vi "Render Inverted Section with Null Array.vi"(8 "Error In":errorcluster) -> (0 "Error Out":errorcluster)   [LabVIEW 2018, in "Tests.lvlib" / "Render.lvlib"]
uses:
  Render.lvlib
  <vilib>/addons/_JKI Toolkits/Caraya/classes/Test/Test.lvclass
  <vilib>/addons/_JKI Toolkits/Caraya/classes/Assert/Assert.lvclass
  src/Toolkit/Toolkit.lvlib
  src/Toolkit/Low-Level/Support/Render to String.vi
  src/Toolkit/Low-Level/Support/Lex String.vi
  src/Toolkit/Data/Null/Null.lvclass
  src/Toolkit/Data/Array/Array.lvclass
  src/Toolkit/Data/Array/Support/From Data.vi
  src/Toolkit/Data/Pair/Pair.lvclass
  src/Toolkit/Data/Pair/Support/From Datum.vi
  src/Toolkit/Low-Level/Context/Compiler.lvclass
  D:/Users/cfield/Code/Field R&D Services/Labstache/src/Toolkit/Data/Datum/Datum.lvclass
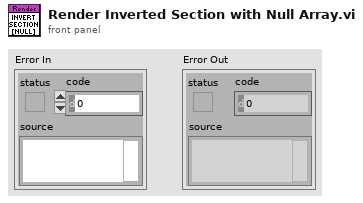
[diagram p1: front panel]
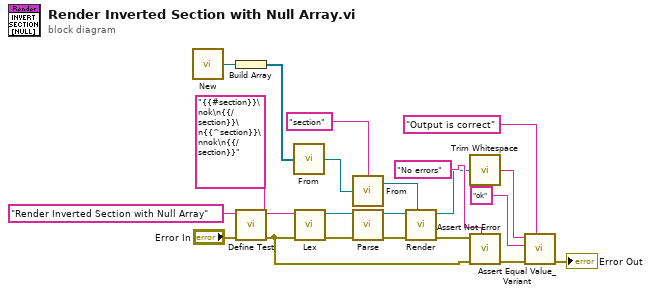
[diagram p0: block diagram]
diagram:
  n1 = call "New.vi"() -> ("Null"=w5:refnum<class "Null.lvclass">)
  n2 = Build Array(w5) -> (w4:refnum<class "Null.lvclass">[])
  n3 = call <vilib>:"Define Test.vi"("error in (no error)"="Error In", "Label (VI Title)"="Render Inverted Section with Null Array") -> ("error out"=w11:errorcluster)  [unwired: 9 in]
  n4 = call-poly "From.vi"("Data"=w4) -> ("Array"=w3:refnum<class "Array.lvclass">)  [unwired: 1 in]
  n5 = call-poly "Lex.vi"("Error In"=w11, "Context In"="{{#section}}\nok\n{{/section}}\n{{^section}}\nnok\n{{/section}}" ("Input")) -> ("Error Out"=w12:errorcluster, "Context Out"=w13:refnum<class "Compiler.lvclass">)  [unwired: 7 in, 1 out]
  n6 = call-poly "From.vi"("Value"=w3, "Key"="section") -> ("Pair"=w1:refnum<class "Pair.lvclass">)
  n7 = call "Parse.vi"("Error In"=w12, "Context In"=w13) -> ("Error Out"=w14:errorcluster, "Context Out"=w10:refnum<class "Compiler.lvclass">)  [unwired: 7 in, 1 out]
  n8 = call-poly "Render.vi"(7:w1, "Error In"=w14, "Context In"=w10) -> ("Error Out"=w15:errorcluster, "Context Out"=w7:refnum<class "Compiler.lvclass">)  [unwired: 6 in, 1 out]
  n9 = call <vilib>:"Trim Whitespace.vi"("string"=w7) -> ("trimmed string"=w6:string)  [unwired: 1 in]
  n10 = call <vilib>:"Assert Not Error.vi"("Label"="No errors", "error in (no error)"=w11, "Not Error?"=w15) -> ("error out"=w18:errorcluster)  [unwired: 8 in]
  n11 = call <vilib>:"Assert Equal Value_Variant.vi"("Label"="Output is correct", "error in (no error)"=w18, "Y"="ok", "X"=w6) -> ("error out"=→"Error Out":errorcluster)  [unwired: 7 in]
